vi "Increment Progress.vi"(11 "Execution UI In":refnum<class "Execution UI V2.lvclass">) -> (2 "Progress (%)":dbl, 3 "Execution UI Out":refnum<class "Execution UI V2.lvclass">)   [LabVIEW 2020, in "Execution UI V2.lvclass"]
uses:
  Execution UI V2.lvclass
  Execution UI V2.lvclass/Execution UI V2.ctl
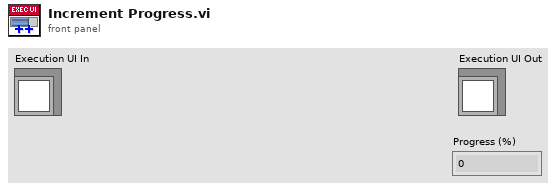
[diagram p1: front panel]
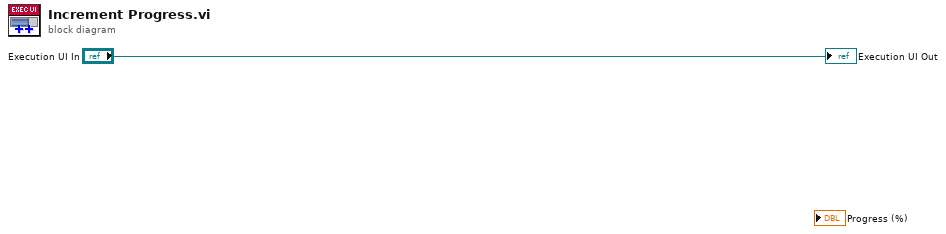
[diagram p0: block diagram]
diagram:
  "Execution UI Out" <- "Execution UI In"
